vi "sine-generate.vi"() -> ()   [LabVIEW 2014]
uses:
  <vilib>/DAQmx/create/channels.llb/DAQmx Create Channel (AO-Voltage-Basic).vi
  <vilib>/DAQmx/configure/timing.llb/DAQmx Timing (Sample Clock).vi
  <vilib>/DAQmx/write.llb/DAQmx Write (Analog Wfm 1Chan NSamp).vi
  <vilib>/measure/NI_MABase.lvlib
  <resource>/objmgr/daqmx.rc
panel:
  in  "error in":errorcluster caption="错误输入"
  in  "amplitude 2":dbl=1.0 format="%#_13g"
  out "signal out":waveform(dbl)(graph) caption="信号输出"
  in  "number of samples":dbl=100.0
  in  "rate":dbl=1000.0
  in  "phase":dbl caption="相位" format="%.2p"
  in  "amplitude":dbl=1.0 caption="幅值" format="%0.2p"
  in  "frequency":dbl=10.0 caption="频率" format="%0.2p"
  in  "stop":bool caption="停止"
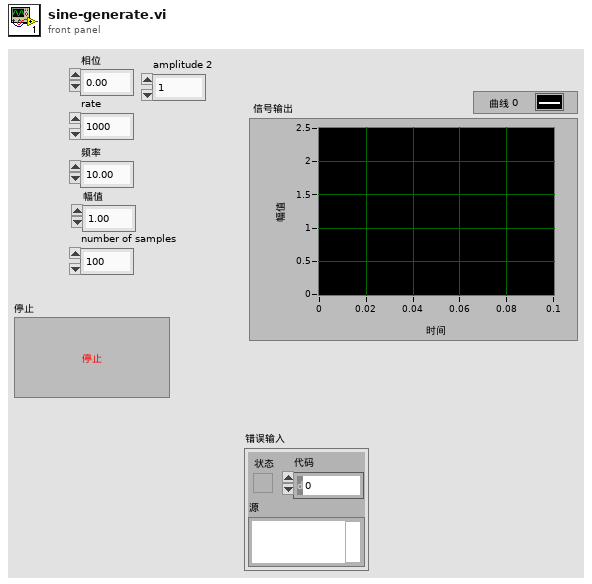
[diagram p1: front panel]
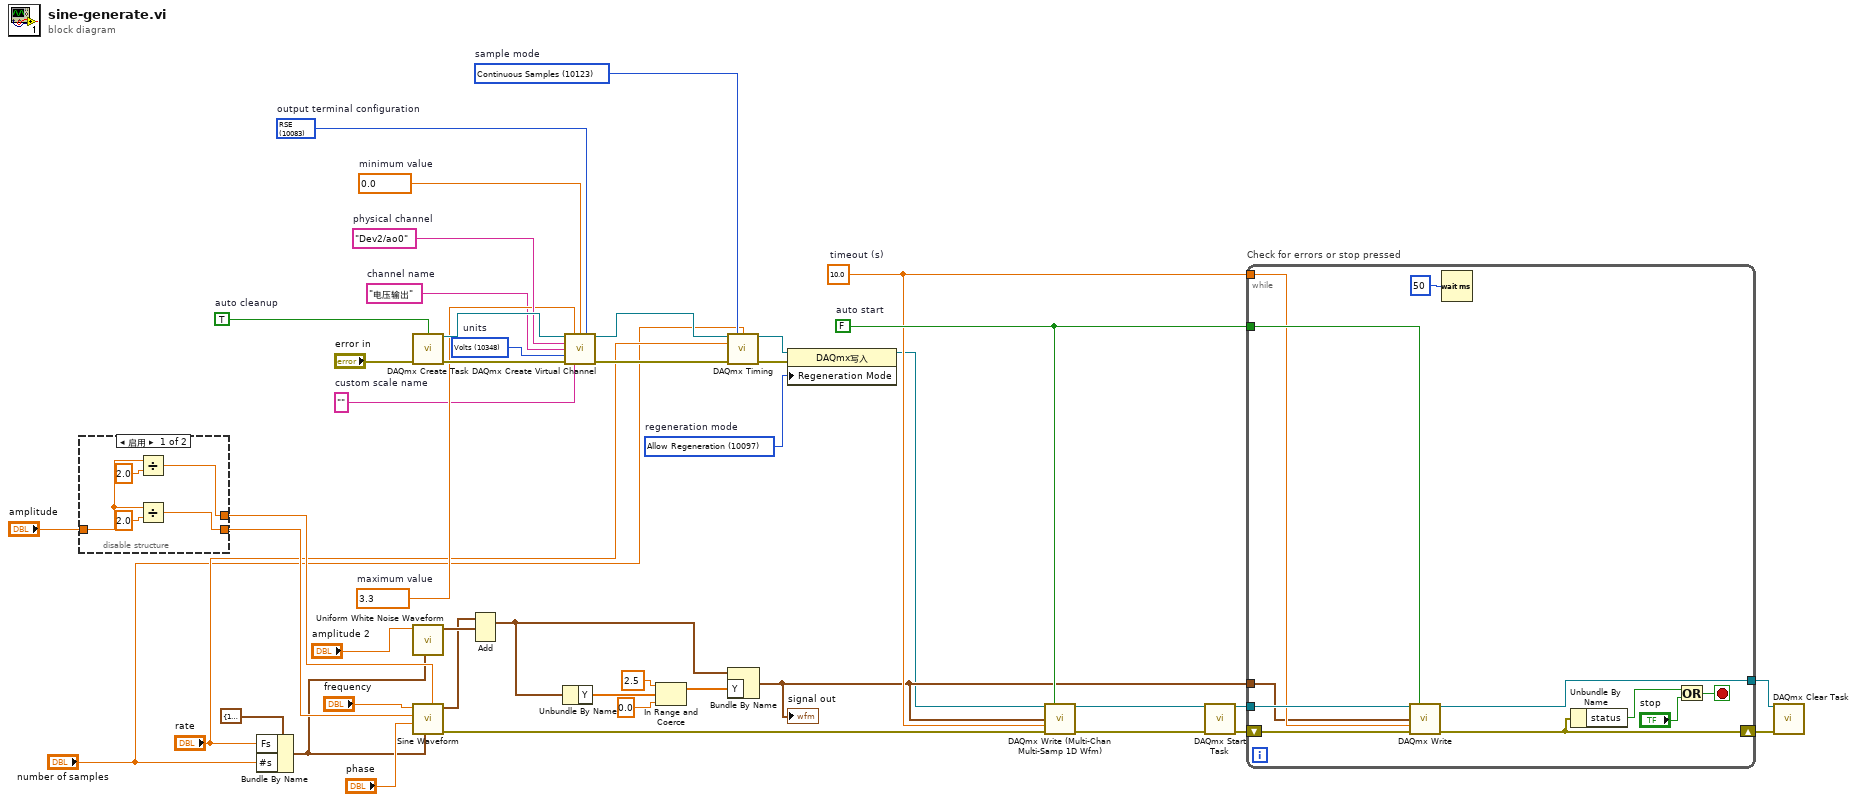
[diagram p0: block diagram]
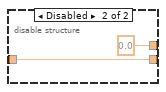
[diagram p2: hidden frame]
diagram:
  w4 = 10097 items=["Allow Regeneration"=10097, "Do Not Allow Regeneration"=10158]  # regeneration mode
  w6 = 10123 items=["Finite Samples"=10178, "Continuous Samples"=10123, "Hardware Timed Single Point"=12522]  # sample mode
  w9 = 10083 items=["Default"=-1, "RSE"=10083, "Differential"=10106, "Pseudodifferential"=12529]  # output terminal configuration
  w10 = 10348 items=["Volts"=10348, "From Custom Scale"=10065]  # units
  w11 = "电压输出"  # channel name
  w13 = ""  # custom scale name
  w14 = 0.0  # minimum value
  w15 = 3.3  # maximum value
  w16 = "Dev2/ao0"  # physical channel
  w18 = TRUE  # auto cleanup
  w37 = 10.0  # timeout (s)
  w38 = FALSE  # auto start
  n1 = disable-structure shown="启用" {
    disable-tunnel: [w50 0.0 ("offset")] -> w33
    disable-tunnel: [w48 w52] -> w32
    disable-tunnel: "amplitude" -> [w47 w52]
    frame Enabled {
      n2 = Divide(x=w47, y=2.0) -> (x/y=w50:dbl)
      n3 = Divide(x=w47, y=2.0) -> (x/y=w48:dbl)
    }
    frame Disabled {
    }
  }
  n4 = Bundle By Name(cluster=cluster{"Fs":dbl, "#s":dbl} {"Fs"=1000.0, "#s"=1000.0} ("sampling info"), "Fs"="rate", "#s"="number of samples") -> (w27:cluster{"Fs":dbl, "#s":dbl})
  n5 = call <vilib>:"DAQmx Create Task.vi"("auto cleanup"=w18, "error in"="error in") -> ("task out"=w17:refnum<k21>, "error out"=w19:errorcluster)  [unwired: 12 in]
  n6 = call <vilib>:"Uniform White Noise Waveform.vi"("sampling info"=w27, "amplitude"="amplitude 2") -> ("signal out"=w29:waveform(dbl))  [unwired: 8 in, 1 out]
  n7 = call <vilib>:"Sine Waveform.vi"("offset"=w33, "sampling info"=w27, "phase"="phase", "amplitude"=w32, "frequency"="frequency") -> ("error out"=w45:errorcluster, "signal out"=w28:waveform(dbl))  [unwired: 5 in]
  n8 = Add(1:w29, 2:w28) -> (0:w22:waveform(dbl))  [unwired: 1 in, 1 out]
  n9 = Unbundle By Name(w22) -> ("Y"=w25:dbl[])
  n10 = call-poly <vilib>:"DAQmx Create Virtual Channel.vi"("task in"=w17, "maximum value"=w15, "minimum value"=w14, "output terminal configuration"=w9, "physical channels"=w16, "name to assign"=w11, "units"=w10, "error in"=w19, "custom scale name"=w13) -> ("task out"=w7:refnum<k21>, "error out"=w12:errorcluster)  [unwired: 5 in]
  n11 = In Range and Coerce(upper limit=2.5, x=w25, lower limit=0.0) -> (coerced(x)=w26:dbl[])  [unwired: 1 out]
  n12 = call-poly <vilib>:"DAQmx Timing.vi"("task/channels in"=w7, "sample mode"=w6, "samples per channel"="number of samples", "rate"="rate", "error in"=w12) -> ("task out"=w5:refnum<k21>, "error out"=w8:errorcluster)  [unwired: 9 in]
  n13 = Bundle By Name(cluster=w22, "Y"=w26) -> (w21:waveform(dbl))
  "signal out" <- w21
  n14 = property class="DAQmx写入"(reference=w5, error in=w8, "Regeneration Mode"=w4) -> (reference out=w3:refnum<k21>)  [unwired: 1 out]
  n15 = call-poly "DAQmx Write (Multi-Chan Multi-Samp 1D Wfm).vi"("task/channels in"=w3, "auto start"=w38, "data"=w21, "timeout"=w37, "error in"=w45) -> ("task out"=w41:refnum<k21>, "error out"=w40:errorcluster)  [unwired: 8 in, 1 out]
  n16 = call <vilib>:"DAQmx Start Task.vi"("task/channels in"=w41, "error in"=w40) -> ("task out"=w43:refnum<k21>, "error out"=w44:errorcluster)  [unwired: 12 in]
  n17 = while "Check for errors or stop pressed" {
    tunnel: [w60] -> w39
    tunnel: w43 -> [w61]
    shift-right: [w57] -> w42
    shift-left: w44 -> [w59]
    tunnel: w38 -> [w55]
    tunnel: w21 -> [w53]
    tunnel: w37 -> [w54]
    stop <- w62 stop-if-true
    n18 = call-poly <vilib>:"DAQmx Write.vi"("task/channels in"=w61, "auto start"=w55, "data"=w53, "timeout"=w54, "error in"=w59) -> ("task out"=w60:refnum<k21>, "error out"=w57:errorcluster)  [unwired: 8 in, 1 out]
    n19 = Wait (ms)(milliseconds to wait=u32 50) -> ()  [unwired: 1 out]
    n20 = Unbundle By Name(w57) -> ("status"=w58:bool)
    n21 = Or(x=w58, y="stop") -> (x .or. y?=w62:bool)
  }
  n22 = call <vilib>:"DAQmx Clear Task.vi"("task in"=w39, "error in"=w42) -> ()  [unwired: 13 in, 1 out]
